vi "Line.vi"(6 "color(black)":u32(colorbox), 8 "error in (no error)":errorcluster, 9 "end point":cluster{"x":i16, "y":i16}, 10 "new position":cluster{"x":i16, "y":i16}, 11 "Tools Paint in":refnum<class "Tools Paint.lvclass">) -> (0 "error out":errorcluster, 2 "new picture":picture, 3 "Tools Paint out":refnum<class "Tools Paint.lvclass">)   [LabVIEW 2021, in "Tools Paint.lvclass"]
uses:
  <resource>/plugins/NIIconEditor/Class/Tools/Tools Paint.lvclass
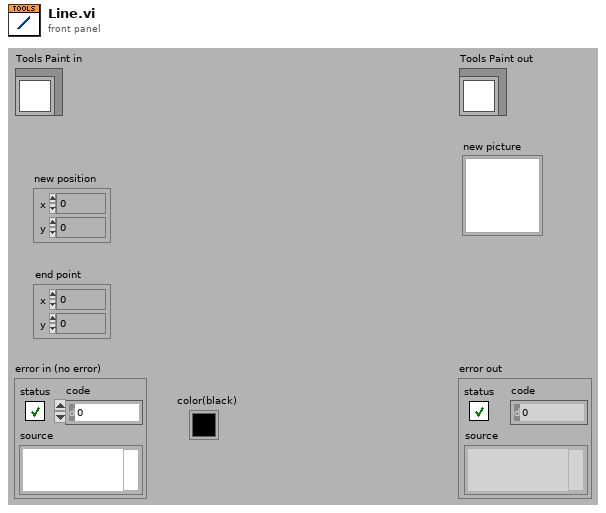
[diagram p1: front panel]
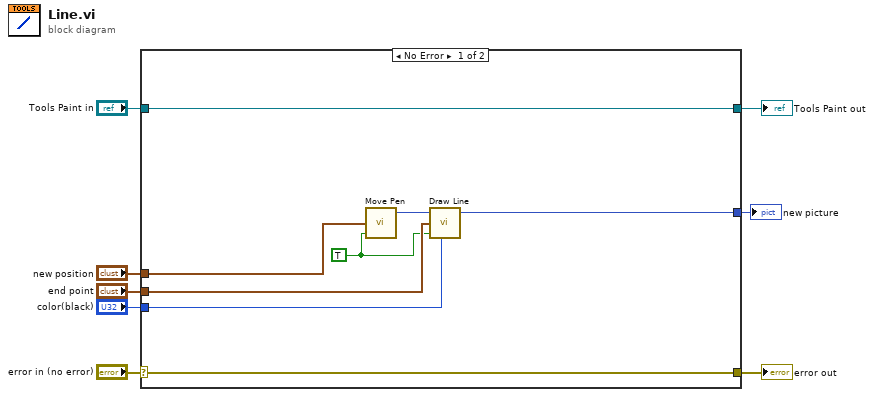
[diagram p0: block diagram]
diagram:
  n1 = case shown="No Error" "error in (no error)" {
    selector: "error in (no error)" -> [w15 w18]
    tunnel: [w15 w18] -> w7
    tunnel: [w16 w17] -> w5
    tunnel: "Tools Paint in" -> [w16 w17]
    tunnel: "end point" -> [w13 _]
    tunnel: "new position" -> [w12 _]
    tunnel: "color(black)" -> [w10 _]
    tunnel: [w9 _] -> w1
    frame No Error {
      w11 = TRUE ("absolute coordinates?(T)")
      n2 = call <vilib>:"Move Pen.vi"("absolute coordinates?(T)"=w11, "new position"=w12) -> ("new picture"=w14:picture)  [unwired: 1 in, 2 out]
      n3 = call <vilib>:"Draw Line.vi"("picture"=w14, "end point"=w13, "absolute coordinates?(T)"=w11, "color(black)"=w10) -> ("new picture"=w9:picture)  [unwired: 1 in, 4 out]
    }
    frame Error {
    }
  }
  "error out" <- w7
  "Tools Paint out" <- w5
  "new picture" <- w1
